vi "Copy Test Vectors.vi"(8 "Error In":errorcluster, 10 "Unit Test Template":path, 11 "Working Dir":path) -> (0 "Error Out":errorcluster)   [LabVIEW 2013, in "VIChallenge.lvlib"]
uses:
  VIChallenge.lvlib
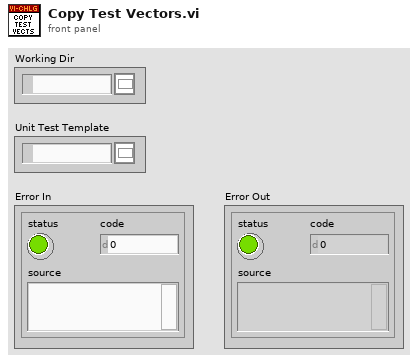
[diagram p1: front panel]
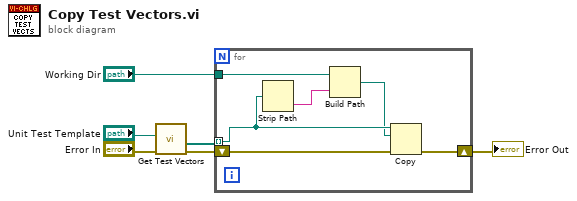
[diagram p0: block diagram]
diagram:
  n1 = call "Get Test Vectors.vi"("Error In"="Error In", "Unit Test Template"="Unit Test Template") -> ("Error Out"=w5:errorcluster, "Test Vector Paths"=w3:path[])  [unwired: 8 in]
  n2 = for {
    tunnel: w3 -> [w12] mode=indexing
    tunnel: "Working Dir" -> [w11]
    shift-right: [w7] -> w6
    shift-left: w5 -> [w8]
    n3 = Strip Path(path=w12) -> (name=w10:string)  [unwired: 1 out]
    n4 = Build Path(base path=w11, name or relative path=w10) -> (appended path=w9:path)
    n5 = Copy(8:w8, 10:w9, 11:w12) -> (0:w7:errorcluster)  [unwired: 2 in, 2 out]
  }
  "Error Out" <- w6
